vi "探测器列表-修改限值.vi"(6 "元素名[]-探测器信息":string[](array[string]), 7 "table名-探测器列表":string, 8 "error in (no error)":errorcluster, 9 "探测器信息":T2, 11 "数据库引用":T1) -> (0 "error out":errorcluster, 3 "connection reference out":T1)   [LabVIEW 2017]
doc: "基本上需要完整的探头属性输入.\n具体需要 网络地址 和 累积限值 / 硬件剂量率限值选择 / 剂量率限值1 / 剂量率限值2 / 报警方式"
uses:
  <vilib>/addons/database/Connection.llb/Conn ObjectReference.ctl
  <vilib>/addons/database/NI_Database_API.lvlib
panel:
  out "Result":string caption="结果"
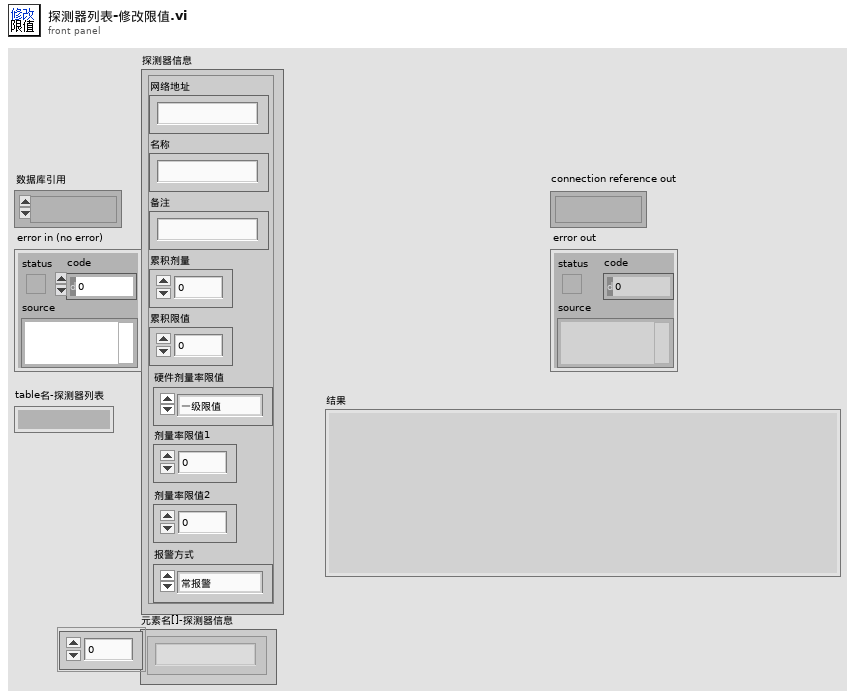
[diagram p1: front panel]
types:
  T1 = typedef "NI_Database_API.lvlib/Conn ObjectReference.ctl" = refnum<k1>
  T2 = typedef "探测器信息.ctl" = cluster{"网络地址":string, "名称":string, "备注":string, "累积剂量":dbl, "累积限值":dbl, "硬件剂量率限值":T3, "剂量率限值1":dbl, "剂量率限值2":dbl, "报警方式":T4}
  T3 = typedef "探头剂量率限值选择.ctl" = enum16{"一级限值", "二级限值"}
  T4 = typedef "报警方式选择.ctl" = enum16{"常报警", "自动静音", "手动静音"}
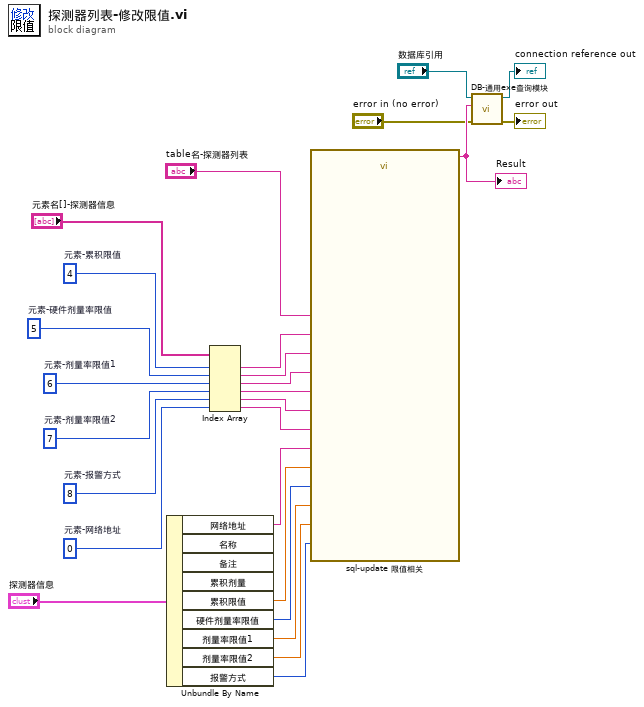
[diagram p0: block diagram]
diagram:
  w12 = 0  # 元素-网络地址
  w13 = 8  # 元素-报警方式
  w17 = 7  # 元素-剂量率限值2
  w18 = 6  # 元素-剂量率限值1
  w20 = 5  # 元素-硬件剂量率限值
  w24 = 4  # 元素-累积限值
  n1 = Unbundle By Name("探测器信息") -> ("网络地址"=w10:string, "累积限值"=w9:dbl, "硬件剂量率限值"=w8:T3, "剂量率限值1"=w7:dbl, "剂量率限值2"=w6:dbl, "报警方式"=w5:T4)  [unwired: 3 out]
  n2 = Index Array(array="元素名[]-探测器信息", index #1=w24, index #2=w20, index #3=w18, index #4=w17, index #5=w13, index #6=w12) -> (element #1=w21:string, element #2=w19:string, element #3=w16:string, element #4=w15:string, element #5=w14:string, element #6=w11:string)
  n3 = call "sql-update 限值相关"("表名-设备表"="table名-探测器列表", "列名-累积限值"=w21, "累积限值"=w9, "列名-硬件剂量率限值选择"=w19, "硬件剂量率限值选择"=w8, "列名-剂量率限值1"=w16, "剂量率限值1"=w7, "列名-剂量率限值2"=w15, "剂量率限值2"=w6, "列名-报警方式"=w14, "报警方式选择"=w5, "列名-网络地址"=w11, "网络地址"=w10) -> ("Result"=w23:string)  [unwired: 13 in, 1 out]
  "Result" <- w23
  n4 = call "DB-通用exe查询模块.vi"("error in (no error)"="error in (no error)", "SQL query"=w23, "数据库连接引用"="数据库引用") -> ("error out"=→"error out":errorcluster, "数据库连接引用out"=→"connection reference out":T1)  [unwired: 4 in, 3 out]
